vi "APS vel.vi"(7 "Wait":cluster{"h_event":u32, "i32_ret":i32}, 8 "error in (no error)":errorcluster caption="错误输入（无错误）", 9 "Vm":dbl, 10 "Option":i32, 11 "Axis_ID":i32) -> (0 "error out":errorcluster caption="错误输出", 3 "function return":i32, 5 "Wait out":cluster{"h_event":u32, "i32_ret":i32})   [LabVIEW 2011, in "APS168.lvlib"]
doc: "I32 FNTYPE APS_vel( I32 Axis_ID, I32 Option, F64 Vm, ASYNCALL *Wait);"
uses:
  APS168.lvlib
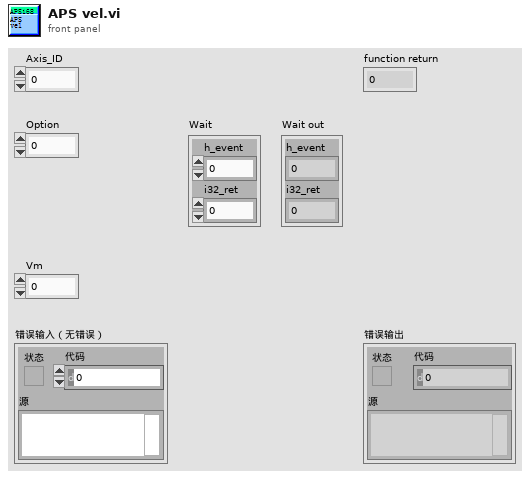
[diagram p1: front panel]
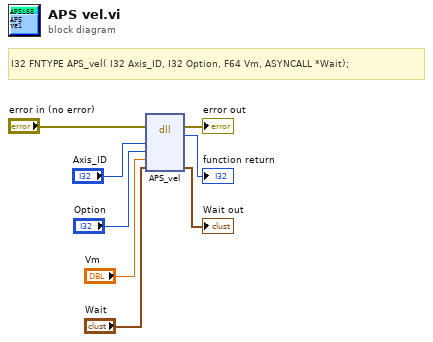
[diagram p0: block diagram]
diagram:
  # "I32 FNTYPE APS_vel( I32 Axis_ID, I32 Option, F64 Vm, ASYNCALL *Wait);"
  n1 = dll-call lib="PTH1Labs E软件ADLINK 204CAPS_1_7_1_LIB line 连续运动204APS168.*" fn="APS_vel"(error in="error in (no error)", "Axis_ID"="Axis_ID", "Option"="Option", "Vm"="Vm", "Wait"="Wait") -> (error out=→"error out":errorcluster, →"function return":i32, "Wait"=→"Wait out":cluster{"h_event":u32, "i32_ret":i32})  [unwired: 5 in, 1 out]
